vi "create context.vi"(8 "error in (no error)":errorcluster, 11 "Communication Manager in":refnum<class "Communication Manager.lvclass">) -> (0 "error out":errorcluster, 3 "Communication Manager out":refnum<class "Communication Manager.lvclass">)   [LabVIEW 2018, in "Communication Manager.lvclass"]
uses:
  Communication Manager.lvclass
  Communication Manager.lvclass/Communication Manager.ctl
  Socket/Socket.lvclass
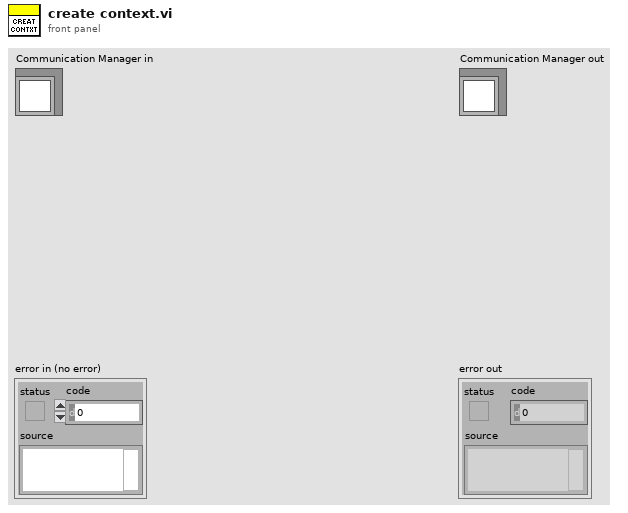
[diagram p1: front panel]
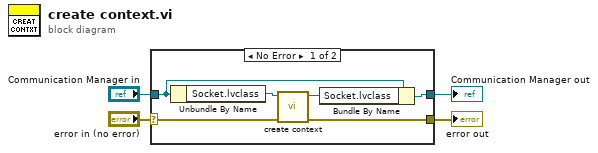
[diagram p0: block diagram]
diagram:
  n1 = case shown="No Error" "error in (no error)" {
    selector: "error in (no error)" -> [w6 w12]
    tunnel: [w5 w12] -> w3
    tunnel: [w9 w11] -> w1
    tunnel: "Communication Manager in" -> [w10 w11]
    frame No Error {
      n2 = Unbundle By Name(w10) -> ("Socket.lvclass"=w8:refnum<class "Socket.lvclass">)
      n3 = call "create context.vi"("error in (no error)"=w6, "Socket in"=w8) -> ("error out"=w5:errorcluster, "Socket out"=w7:refnum<class "Socket.lvclass">)  [unwired: 8 in]
      n4 = Bundle By Name(cluster=w10, "Socket.lvclass"=w7) -> (w9:refnum<class "Communication Manager.lvclass">)
    }
    frame Error {
    }
  }
  "error out" <- w3
  "Communication Manager out" <- w1
